vi "structure-tunnel-wire-bends.vi"() -> ()   [LabVIEW 2025]
panel:
  out "Numeric 2":i32
  in  "Numeric":i32
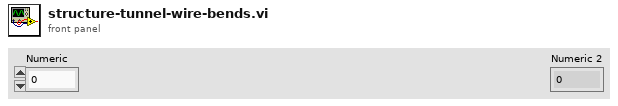
[diagram p1: front panel]
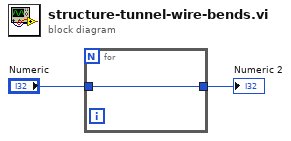
[diagram p0: block diagram]
diagram:
  n1 = for {
    tunnel: "Numeric" -> [w3]
    tunnel: [w3] -> w2
  }
  "Numeric 2" <- w2
